vi "Auto Get Configuration Info.vi"(8 "error in (no error)":errorcluster, 11 "Data Cluster in":T1) -> (0 "error out":errorcluster, 3 "Data Cluster out":T1)   [LabVIEW 2017]
uses:
  controls/Auto UI Data.ctl
  controls/Configuration Details.ctl
  Database/Controls/DB Options.ctl
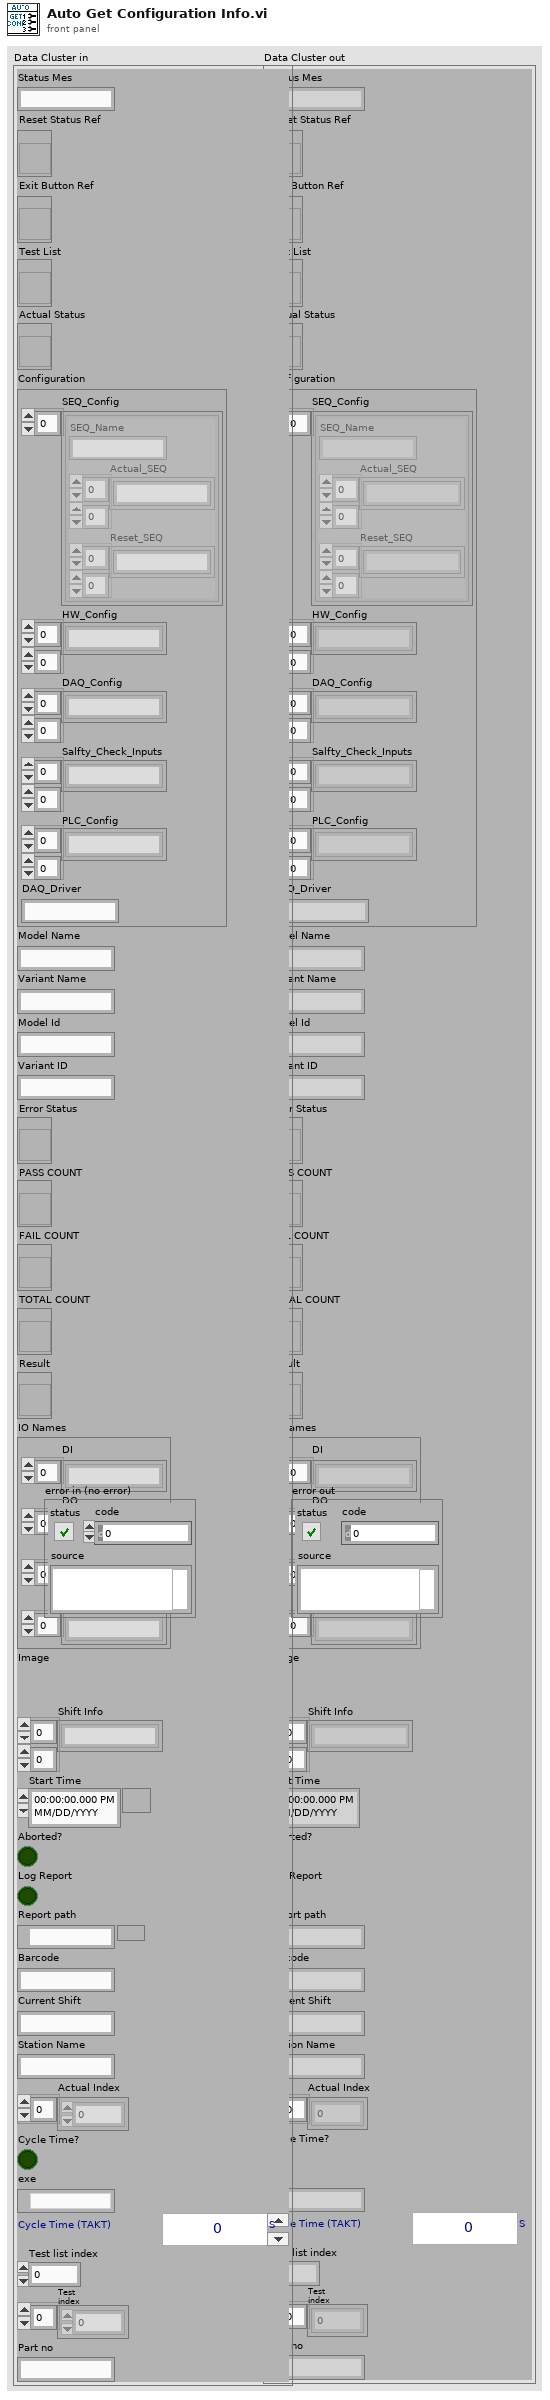
[diagram p1: front panel]
types:
  T1 = typedef "Auto UI Data.ctl" = cluster{"Status Mes":string, "Reset Status Ref":refnum<vi>, "Exit Button Ref":refnum<vi>, "Test List":refnum<vi>, "Actual Status":refnum<vi>, "Configuration":T2, "Model Name":string, "Variant Name":string, "Model Id":string, "Variant ID":string, "Error Status":refnum<vi>, "PASS COUNT":refnum<vi>, "FAIL COUNT":refnum<vi>, "TOTAL COUNT":refnum<vi>, "Result":refnum<vi>, "IO Names":cluster{"DI":string[], "DO":string[], "AI":string[], "AO":string[]}, "Image":T3, "Shift Info":string[][], "Start Time":timestamp, "Aborted?":bool, "Log Report":bool, "Report path":path, "Barcode":string, "Current Shift":string, "Station Name":string, "Actual Index":i32[], "Cycle Time?":bool, "exe":path, "Cycle Time (TAKT)":u16, "Test list index":u32, "Test index":u32[], "Part no":string}
  T2 = typedef "Configuration Details.ctl" = cluster{"SEQ_Config":cluster{"SEQ_Name":string, "Actual_SEQ":string[][], "Reset_SEQ":string[][]}[], "HW_Config":string[][], "DAQ_Config":string[][], "Salfty_Check_Inputs":string[][], "PLC_Config":string[][], "DAQ_Driver":string}
  T3 = typedef "IMAQ Image.ctl" = refnum<image>
  T4 = typedef "DB Options.ctl" = enum16{"Select", "Execute", "Special Q", "Insert", "Update", "Delete", "Open", "Close"}
  T5 = cluster{"SEQ_Name":string, "Actual_SEQ":string[][], "Reset_SEQ":string[][]}
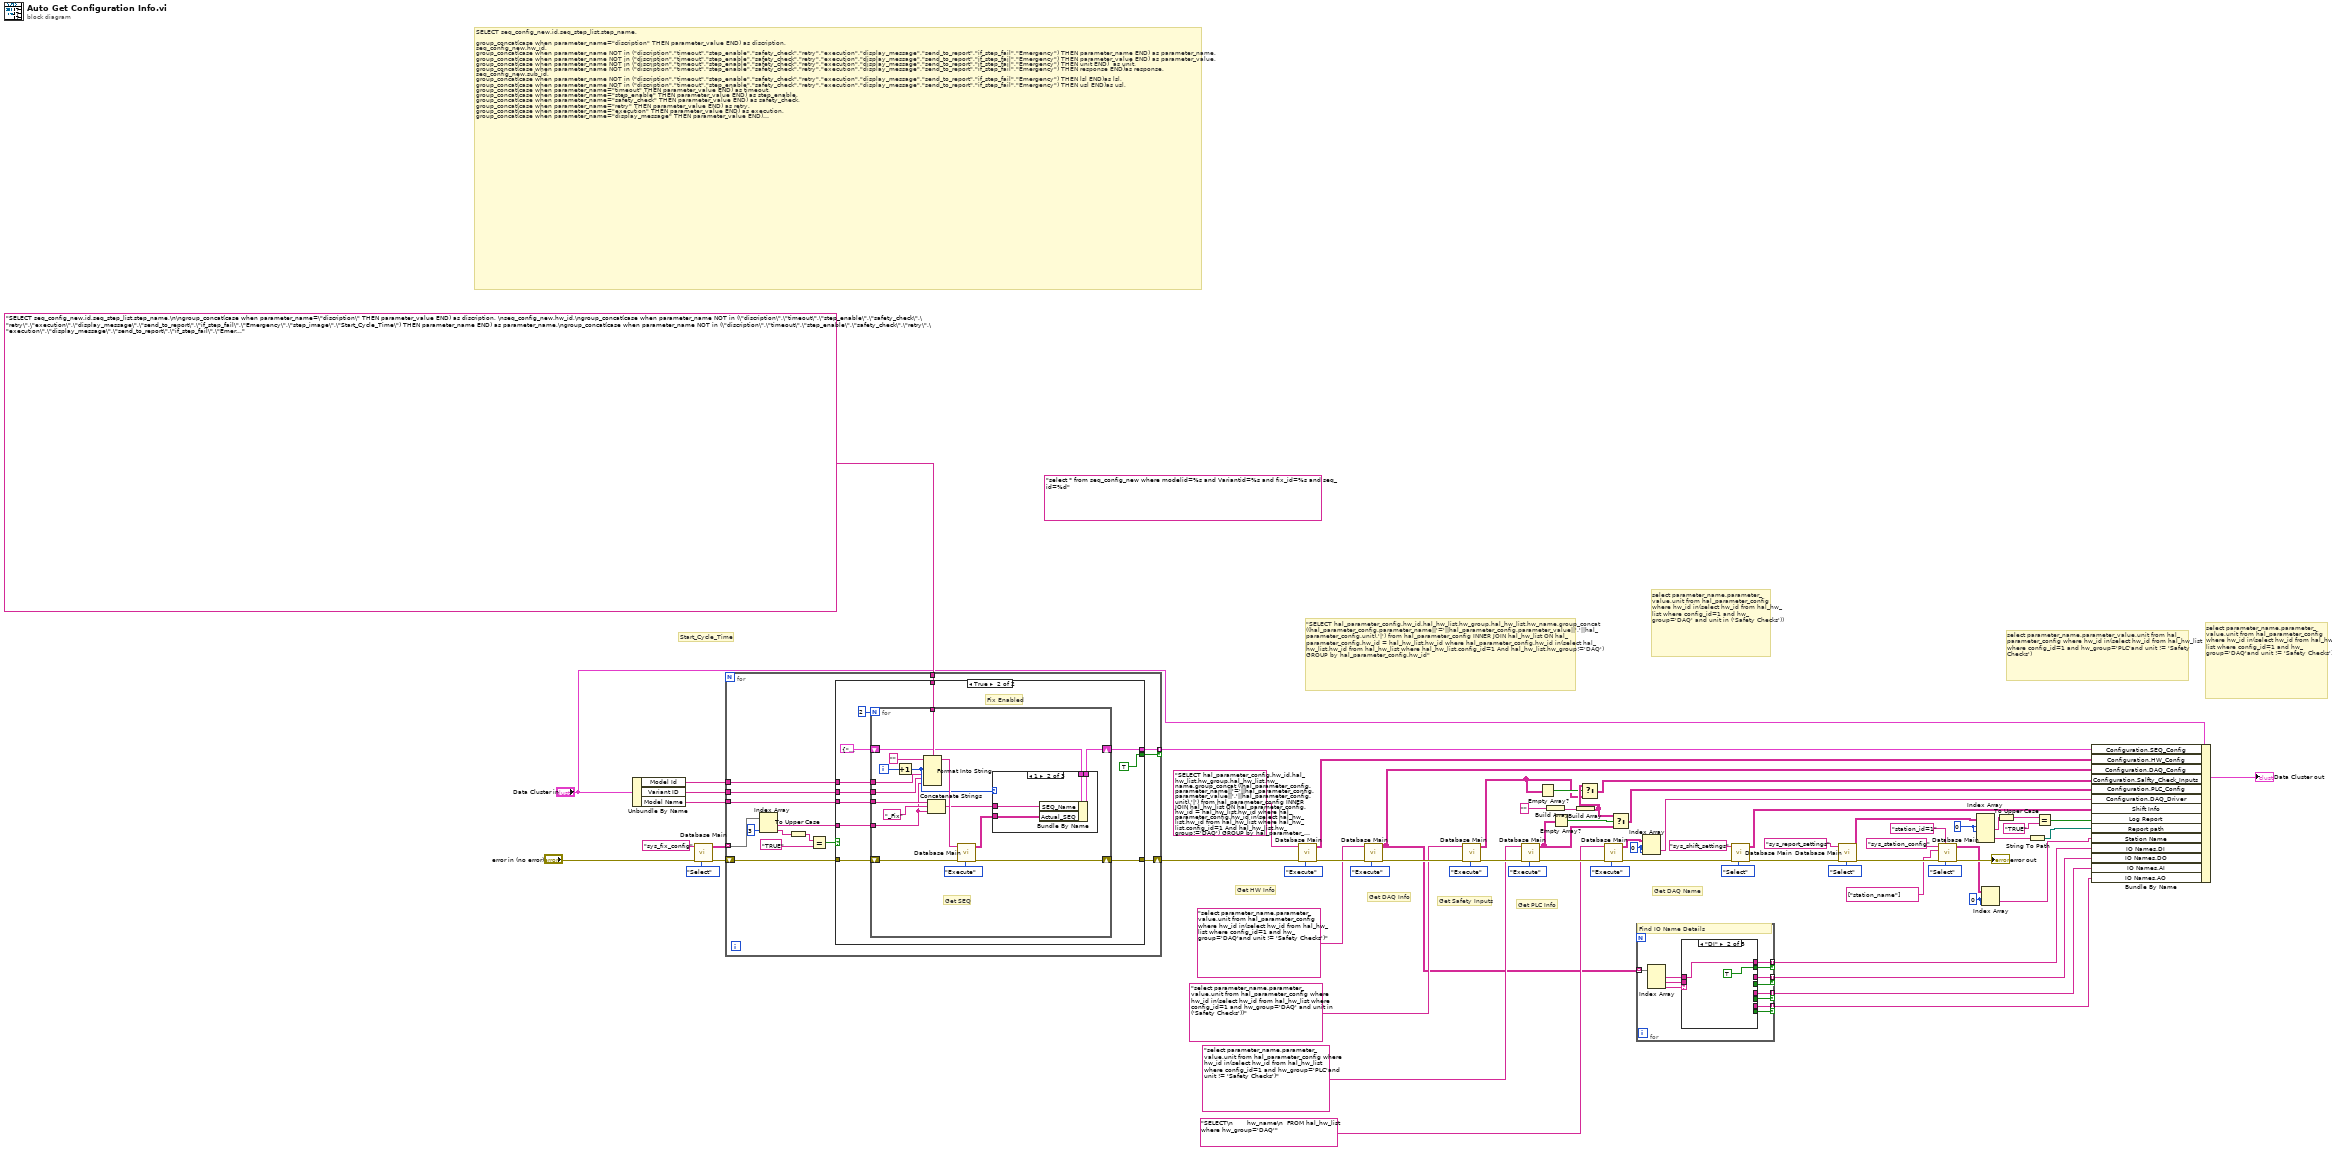
[diagram p0: block diagram]
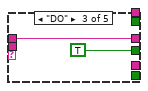
[diagram p3: hidden frame]
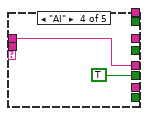
[diagram p4: hidden frame]
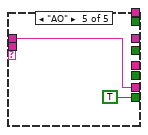
[diagram p5: hidden frame]
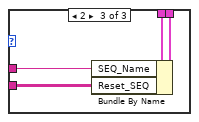
[diagram p8: hidden frame]
diagram:
  w3 = 0 ("index (row)")
  w16 = 0 ("index (row)")
  (unwired) "select * from seq_config_new where modelid=%s and Variantid=%s and fix_id=%s and seq_id=%d" ("Where")
  w40 = 0 ("index (row)")
  # "Start_Cycle_Time"
  # "SELECT seq_config_new.id,seq_step_list.step_name,\n\ngroup_concat(case when parameter_name=\"discription\" THEN parameter_value END) as discription, \nseq_config_new.hw_id,\ngroup_concat(case when parameter_name NOT in (\"discription\",\"timeout\",\"step_enable\",\"safety_check\",\"retry\",\"execution\",\"display_message\",\"send_to_report\",\"if_step_fail\",\"Emergency\") THEN parameter_name END) as parameter_name,\ngroup_concat(case when parameter_name NOT in (\"discription\",\"timeout\",\"step_enable\",\"safety_check\",\"retry\",\"execution\",\"display_message\",\"send_to_report\",\"if_step_fail\",\"Emergency\") THEN parameter_value END) as parameter_value,\ngroup_concat(case when parameter_name NOT in (\"discription\",\"timeout\",\"step_enable\",\"safety_check\",\"retry\",\"execution\",\"display_message\",\"send_to_report\",\"if_step_fail\",\"Emergency\") THEN unit END)  as unit,\ngroup_concat(case when parameter_name NOT in (\"discription\",\"timeout\",\"step_enable\",\"safety_check\",\"retry\",\"execution\",\"display_message\",\"send_to_report\",\"if_step_fail\",\"Emergency\") THEN response END)as response,\nseq_config_new.sub_id,\ngroup_concat(case when parameter_name NOT in (\"discription\",\"timeout\",\"step_enable\",\"safety_check\",\"retry\",\"execution\",\"display_message\",\"send_to_report\",\"if_step_fail\",\"Emergency\") THEN lsl END)as lsl,\ngroup_concat(case when parameter_name NOT in (\"discription\",\"timeout\",\"step_enable\",\"safety_check\",\"retry\",\"execution\",\"display_message\",\"send_to_report\",\"if_step_fail\",\"Emergency\") THEN usl END)as usl,\ngroup_concat(case when parameter_name=\"timeout\" THEN parameter_value END) as timeout,\ngroup_concat(case when parameter_name=\"step_enable\" THEN parameter_value END) as step_enable,\ngroup_concat(case when parameter_name=\"safety_check\" THEN parameter_value END) as safety_check,\ngroup_concat(case when parameter_name=\"retry\" THEN parameter_value END) as retry,\ngroup_concat(case when parameter_name=\"execution\" THEN parameter_value END) as execution,\ngroup_concat(case when parameter_name=\"display_message\" THEN parameter_value END) as display_message,\ngroup_concat(case when parameter_name=\"send_to_report\" THEN parameter_value END) as send_to_report,\ngroup_concat(case when parameter_name=\"if_step_fail\" THEN parameter_value END) as if_step_fail,\ngroup_concat(case when parameter_name=\"Emergency\" THEN parameter_value END) as Emergency\n\nfrom seq_config_new\n\nINNER JOIN seq_step_list ON seq_config_new.step_name_id = seq_step_list.step_id \n\nwhere seq_config_new.seq_id= (SELECT seq_id FROM seq_list where model_id=1 and seq_name=\"Actual SEQ\") and seq_config_new.fix_id=2 and modelid=3 and variantid=3\n   \nGROUP by \nseq_config_new.id,\nseq_config_new.sub_id"
  # "Get DAQ Name"
  # "Get PLC Info"
  # "Get Safety Inputs"
  # "Get DAQ Info"
  # "select parameter_name,parameter_value,unit from hal_parameter_config where hw_id in(select hw_id from hal_hw_list where config_id=1 and hw_group='DAQ'and unit != 'Safety Checks')"
  # "select parameter_name,parameter_value,unit from hal_parameter_config where hw_id in(select hw_id from hal_hw_list where config_id=1 and hw_group='PLC'and unit != 'Safety Checks')"
  # "select parameter_name,parameter_value,unit from hal_parameter_config where hw_id in(select hw_id from hal_hw_list where config_id=1 and hw_group='DAQ' and unit in ('Safety Checks'))"
  # "Get HW Info"
  # "\"SELECT hal_parameter_config.hw_id,hal_hw_list.hw_group,hal_hw_list.hw_name,group_concat ((hal_parameter_config.parameter_name||'='||hal_parameter_config.parameter_value||','||hal_parameter_config.unit),'|') from hal_parameter_config INNER JOIN hal_hw_list ON hal_parameter_config.hw_id = hal_hw_list.hw_id where hal_parameter_config.hw_id in(select hal_hw_list.hw_id from hal_hw_list where hal_hw_list.config_id=1 And hal_hw_list.hw_group!='DAQ') GROUP by hal_parameter_config.hw_id\""
  n1 = Unbundle By Name("Data Cluster in") -> ("Model Id"=w66:string, "Variant ID"=w68:string, "Model Name"=w60:string)
  n2 = call "Database Main.vi"("Option"=DB_Options."Select", "error in (no error)"="error in (no error)", "table Name/Query"="sys_fix_config") -> ("error out"=w69:errorcluster, "Data"=w65:string[][])  [unwired: 6 in, 1 out]
  n3 = for {
    tunnel: w65 -> [w84] mode=indexing
    tunnel: w66 -> [w83]
    tunnel: "SELECT seq_config_new.id,seq_step_list.step_name,\n\ngroup_concat(case when parameter_name=\"discription\" THEN parameter_value END) as discription, \nseq_config_new.hw_id,\ngroup_concat(case when parameter_name NOT in (\"discription\",\"timeout\",\"step_enable\",\"safety_check\",\"retry\",\"execution\",\"display_message\",\"send_to_report\",\"if_step_fail\",\"Emergency\",\"step_image\",\"Start_Cycle_Time\") THEN parameter_name END) as parameter_name,\ngroup_concat(case when parameter_name NOT in (\"discription\",\"timeout\",\"step_enable\",\"safety_check\",\"retry\",\"execution\",\"display_message\",\"send_to_report\",\"if_step_fail\",\"Emergency\",\"step_image\",\"Start_Cycle_Time\") THEN parameter_value END) as parameter_value,\ngroup_concat(case when parameter_name NOT in (\"discription\",\"timeout\",\"step_enable\",\"safety_check\",\"retry\",\"execution\",\"display_message\",\"send_to_report\",\"if_step_fail\",\"Emergency\",\"step_image\",\"Start_Cycle_Time\") THEN unit END)  as unit,\ngroup_concat(case when parameter_name NOT in (\"discription\",\"timeout\",\"step_enable\",\"safety_check\",\"retry\",\"execution\",\"display_message\",\"send_to_report\",\"if_step_fail\",\"Emergency\",\"step_image\",\"Start_Cycle_Time\") THEN response END)as response,\nseq_config_new.sub_id,\ngroup_concat(case when parameter_name NOT in (\"discription\",\"timeout\",\"step_enable\",\"safety_check\",\"retry\",\"execution\",\"display_message\",\"send_to_report\",\"if_step_fail\",\"Emergency\",\"step_image\",\"Start_Cycle_Time\") THEN lsl END)as lsl,\ngroup_concat(case when parameter_name NOT in (\"discription\",\"timeout\",\"step_enable\",\"safety_check\",\"retry\",\"execution\",\"display_message\",\"send_to_report\",\"if_step_fail\",\"Emergency\",\"step_image\",\"Start_Cycle_Time\") THEN usl END)as usl,\ngroup_concat(case when parameter_name=\"timeout\" THEN parameter_value END) as timeout,\ngroup_concat(case when parameter_name=\"step_enable\" THEN parameter_value END) as step_enable,\ngroup_concat(case when parameter_name=\"safety_check\" THEN parameter_value END) as safety_check,\ngroup_concat(case when parameter_name=\"retry\" THEN parameter_value END) as retry,\ngroup_concat(case when parameter_name=\"execution\" THEN parameter_value END) as execution,\ngroup_concat(case when parameter_name=\"display_message\" THEN parameter_value END) as display_message,\ngroup_concat(case when parameter_name=\"send_to_report\" THEN parameter_value END) as send_to_report,\ngroup_concat(case when parameter_name=\"if_step_fail\" THEN parameter_value END) as if_step_fail,\ngroup_concat(case when parameter_name=\"Emergency\" THEN parameter_value END) as Emergency,\ngroup_concat(case when parameter_name NOT in (\"discription\",\"timeout\",\"step_enable\",\"safety_check\",\"retry\",\"execution\",\"display_message\",\"send_to_report\",\"if_step_fail\",\"Emergency\",\"step_image\",\"Start_Cycle_Time\") THEN testname END)  as testname,\ngroup_concat(case when parameter_name NOT in (\"discription\",\"timeout\",\"step_enable\",\"safety_check\",\"retry\",\"execution\",\"display_message\",\"send_to_report\",\"if_step_fail\",\"Emergency\",\"step_image\",\"Start_Cycle_Time\") THEN showtest END)  as showtest,\ngroup_concat(case when parameter_name=\"step_image\" THEN parameter_value END) as step_image,\ngroup_concat(case when parameter_name=\"Start_Cycle_Time\" THEN parameter_value END) as Start_Cycle_Time\n\nfrom seq_config_new\n\nINNER JOIN seq_step_list ON seq_config_new.step_name_id = seq_step_list.step_id \n\nwhere seq_config_new.seq_id= (SELECT seq_id FROM seq_list where model_id=1 and seq_id=%d) and modelid=%s and variantid=%s and seq_config_new.fix_id=%s\n   \nGROUP by \nseq_config_new.id,\nseq_config_new.sub_id" ("Where") -> [w82]
    tunnel: w68 -> [w81]
    shift-right: [w79] -> w56
    shift-left: w69 -> [w80]
    tunnel: w60 -> [w78]
    tunnel: [w76] -> w58 mode=indexing if=w70
    n4 = Index Array(array=w84, index #2=3 ("index")) -> (element #1=w77:string, element #2=w74:string)  [unwired: 1 in]
    n5 = To Upper Case(1:w74) -> (0:w72:string)
    n6 = Equal?(x=w72, y="TRUE") -> (x = y?=w71:bool)
    n7 = case shown="True" w71 {
      tunnel: w83 -> [_ w96]
      tunnel: w82 -> [_ w95]
      tunnel: w81 -> [_ w94]
      tunnel: w80 -> [w85 w93]
      tunnel: [w85 w92] -> w79
      tunnel: w78 -> [_ w89]
      tunnel: w77 -> [_ w88]
      tunnel: [_ w87] -> w76
      tunnel: [_ TRUE] -> w70
      frame False {
        # "Fix Disabled"
      }
      frame True {
        # "Fix Enabled"
        n8 = for {
          N: 2 -> [_]
          tunnel: w96 -> [w99]
          tunnel: w95 -> [w112]
          tunnel: w94 -> [w98]
          tunnel: w88 -> [w97]
          shift-right: [w107] -> w92
          shift-left: w93 -> [w108]
          tunnel: w89 -> [w104]
          shift-right: [w105] -> w87
          shift-left: T5 {"SEQ_Name"="", "Actual_SEQ"=[], "Reset_SEQ"=[]} ("Configuration") -> [w106]
          i -> [w111]
          # "Get SEQ"
          n9 = Increment(x=w111) -> (x+1=w100:i32)
          n10 = Format Into String(format string=w112, initial string="", w100, w99, w98, w97) -> (resulting string=w109:string)  [unwired: 1 in, 1 out]
          n11 = Concatenate Strings(w104, "_Fix" ("string"), w97) -> (w102:string)
          n12 = call "Database Main.vi"("Option"=DB_Options."Execute", "error in (no error)"=w108, "table Name/Query"=w109) -> ("error out"=w107:errorcluster, "Data"=w101:string[][])  [unwired: 6 in, 1 out]
          n13 = case shown="1" w100 {
            tunnel: w106 -> [w114 w118 w122]
            tunnel: [w114 w117 w121] -> w105
            tunnel: w102 -> [_ w116 w120]
            tunnel: w101 -> [_ w115 w119]
            frame 0, Default {
            }
            frame 1 {
              n14 = Bundle By Name(cluster=w118, "SEQ_Name"=w116, "Actual_SEQ"=w115) -> (w117:T5)
            }
            frame 2 {
              n15 = Bundle By Name(cluster=w122, "SEQ_Name"=w120, "Reset_SEQ"=w119) -> (w121:T5)
            }
          }
        }
      }
    }
  }
  n16 = call "Database Main.vi"("Option"=DB_Options."Execute", "error in (no error)"=w56, "table Name/Query"="SELECT hal_parameter_config.hw_id,hal_hw_list.hw_group,hal_hw_list.hw_name,group_concat ((hal_parameter_config.parameter_name||'='||hal_parameter_config.parameter_value||','||hal_parameter_config.unit),'|') from hal_parameter_config INNER JOIN hal_hw_list ON hal_parameter_config.hw_id = hal_hw_list.hw_id where hal_parameter_config.hw_id in(select hal_hw_list.hw_id from hal_hw_list where hal_hw_list.config_id=1 And hal_hw_list.hw_group!='DAQ') GROUP by hal_parameter_config.hw_id") -> ("error out"=w52:errorcluster, "Data"=w54:string[][])  [unwired: 6 in, 1 out]
  n17 = call "Database Main.vi"("Option"=DB_Options."Execute", "error in (no error)"=w52, "table Name/Query"="select parameter_name,parameter_value,unit from hal_parameter_config where hw_id in(select hw_id from hal_hw_list where config_id=1 and hw_group='DAQ'and unit != 'Safety Checks')") -> ("error out"=w49:errorcluster, "Data"=w38:string[][])  [unwired: 6 in, 1 out]
  n18 = call "Database Main.vi"("Option"=DB_Options."Execute", "error in (no error)"=w49, "table Name/Query"="select parameter_name,parameter_value,unit from hal_parameter_config where hw_id in(select hw_id from hal_hw_list where config_id=1 and hw_group='DAQ' and unit in ('Safety Checks'))") -> ("error out"=w46:errorcluster, "Data"=w26:string[][])  [unwired: 6 in, 1 out]
  n19 = call "Database Main.vi"("Option"=DB_Options."Execute", "error in (no error)"=w46, "table Name/Query"="select parameter_name,parameter_value,unit from hal_parameter_config where hw_id in(select hw_id from hal_hw_list where config_id=1 and hw_group='PLC'and unit != 'Safety Checks')") -> ("error out"=w43:errorcluster, "Data"=w30:string[][])  [unwired: 6 in, 1 out]
  n20 = Empty Array?(array=w26) -> (empty?=w27:bool)
  n21 = Build Array("") -> (w32:string[])
  n22 = Empty Array?(array=w30) -> (empty?=w31:bool)
  n23 = Build Array(w32) -> (w28:string[][])
  n24 = Select(t=w28, s=w27, f=w26) -> (s? t:f=w25:string[][])
  n25 = call "Database Main.vi"("Option"=DB_Options."Execute", "error in (no error)"=w43, "table Name/Query"="SELECT\n       hw_name\n  FROM hal_hw_list where hw_group='DAQ'") -> ("error out"=w24:errorcluster, "Data"=w41:string[][])  [unwired: 6 in, 1 out]
  n26 = Select(t=w28, s=w31, f=w30) -> (s? t:f=w29:string[][])
  n27 = for {
    tunnel: w38 -> [w134] mode=indexing
    tunnel: [w130] -> w37 mode=indexing if=w129
    tunnel: [w128] -> w36 mode=indexing if=w127
    tunnel: [w126] -> w35 mode=indexing if=w125
    tunnel: [w124] -> w34 mode=indexing if=w123
    # "Find IO Name Details"
    n28 = Index Array(array=w134) -> (element #1=w131:string, element #2=w132:string, element #3=w133:string)  [unwired: 3 in]
    n29 = case shown="\"DI\"" w133 {
      tunnel: w132 -> [_ _ _ _ _]
      tunnel: w131 -> [_ w135 w137 w140 w142]
      tunnel: [_ w135 _ _ _] -> w130
      tunnel: [_ TRUE _ _ _] -> w129
      tunnel: [_ _ w137 _ _] -> w128
      tunnel: [_ _ TRUE _ _] -> w127
      tunnel: [_ _ _ w140 _] -> w126
      tunnel: [_ _ _ TRUE _] -> w125
      tunnel: [_ _ _ _ w142] -> w124
      tunnel: [_ _ _ _ TRUE] -> w123
      frame Default {
      }
      frame "DI" {
      }
      frame "DO" {
      }
      frame "AI" {
      }
      frame "AO" {
      }
    }
  }
  n30 = Index Array(array=w41, index (row)=w40, index (col)=w40) -> (element=w39:string)
  n31 = call "Database Main.vi"("Option"=DB_Options."Select", "error in (no error)"=w24, "table Name/Query"="sys_shift_settings") -> ("error out"=w18:errorcluster, "Data"=w22:string[][])  [unwired: 6 in, 1 out]
  n32 = call "Database Main.vi"("Option"=DB_Options."Select", "error in (no error)"=w18, "table Name/Query"="sys_report_settings") -> ("error out"=w8:errorcluster, "Data"=w17:string[][])  [unwired: 6 in, 1 out]
  n33 = call "Database Main.vi"("Option"=DB_Options."Select", "Where"="station_id=1", "error in (no error)"=w8, "Column Name"=string[] ["station_name"], "table Name/Query"="sys_station_config") -> ("error out"=→"error out":errorcluster, "Data"=w5:string[][])  [unwired: 4 in, 1 out]
  n34 = Index Array(array=w17, index (row) #1=w16, index (col) #1=w16) -> (element #1=w15:string, element #2=w11:string)  [unwired: 2 in]
  n35 = Index Array(array=w5, index (row)=w3, index (col)=w3) -> (element=w4:string)
  n36 = To Upper Case(1:w15) -> (0:w12:string)
  n37 = String To Path(string=w11) -> (path=w10:path)
  n38 = Equal?(x=w12, y="TRUE") -> (x = y?=w14:bool)
  n39 = Bundle By Name(cluster="Data Cluster in", "Configuration.SEQ_Config"=w58, "Configuration.HW_Config"=w54, "Configuration.DAQ_Config"=w38, "Configuration.Salfty_Check_Inputs"=w25, "Configuration.PLC_Config"=w29, "Configuration.DAQ_Driver"=w39, "Shift Info"=w22, "Log Report"=w14, "Report path"=w10, "Station Name"=w4, "IO Names.DI"=w37, "IO Names.DO"=w36, "IO Names.AI"=w35, "IO Names.AO"=w34) -> (→"Data Cluster out":T1)
